vi "FPGA Reference - Open.vi"(8 "error in":errorcluster, 11 "FPGA resource name":T1) -> (0 "error out":errorcluster)   [LabVIEW 2024, in "FPGA Interface.lvlib"]
uses:
  FPGA Interface.lvlib
  <vilib>/userDefined/High Color/nirio_resource_hc.ctl
  FPGA Ref Action.ctl
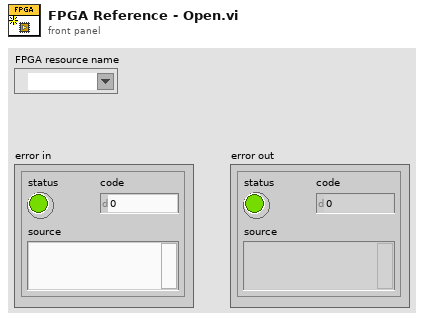
[diagram p1: front panel]
types:
  T1 = typedef "nirio_resource_hc.ctl" = tag
  T2 = typedef "FPGA Interface.lvlib/FPGA Ref Action.ctl" = enum16{"Open Ref", "Get Ref", "Close Ref"}
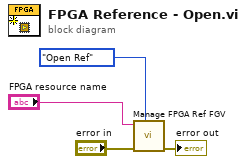
[diagram p0: block diagram]
diagram:
  n1 = call "Manage FPGA Ref FGV.vi"("FPGA Action"=FPGA_Ref_Action."Open Ref", "error in"="error in", "FPGA resource name"="FPGA resource name") -> ("error out"=→"error out":errorcluster)  [unwired: 7 in, 1 out]
